vi "AlignDUT.vi"() -> ()   [LabVIEW 2018]
uses:
  <vilib>/userdefined/High Color/IMAQdx.ctl
  <vilib>/vision/driver/NI_Vision_Acquisition_Software.lvlib
  <vilib>/vision/NI_Vision_Development_Module.lvlib
panel:
  out "Average Length Between Fiducials":dbl format="%0.2f"
  in  "Number of Iterations":i32=50
  in  "Sensor Type":string(combo)="R0Hamamatsu"
  in  "Second Move OK?":bool
  in  "Second Fiducial OK?":bool
  in  "Second Fiducial in View?":bool
  in  "First Move OK?":bool
  in  "First Fiducial OK?":bool
  out "Pattern Matched Image":T1(plugin-control) caption="Template Image"
  out "Image Out":T1(plugin-control)
  in  "Fiducial 1":bool
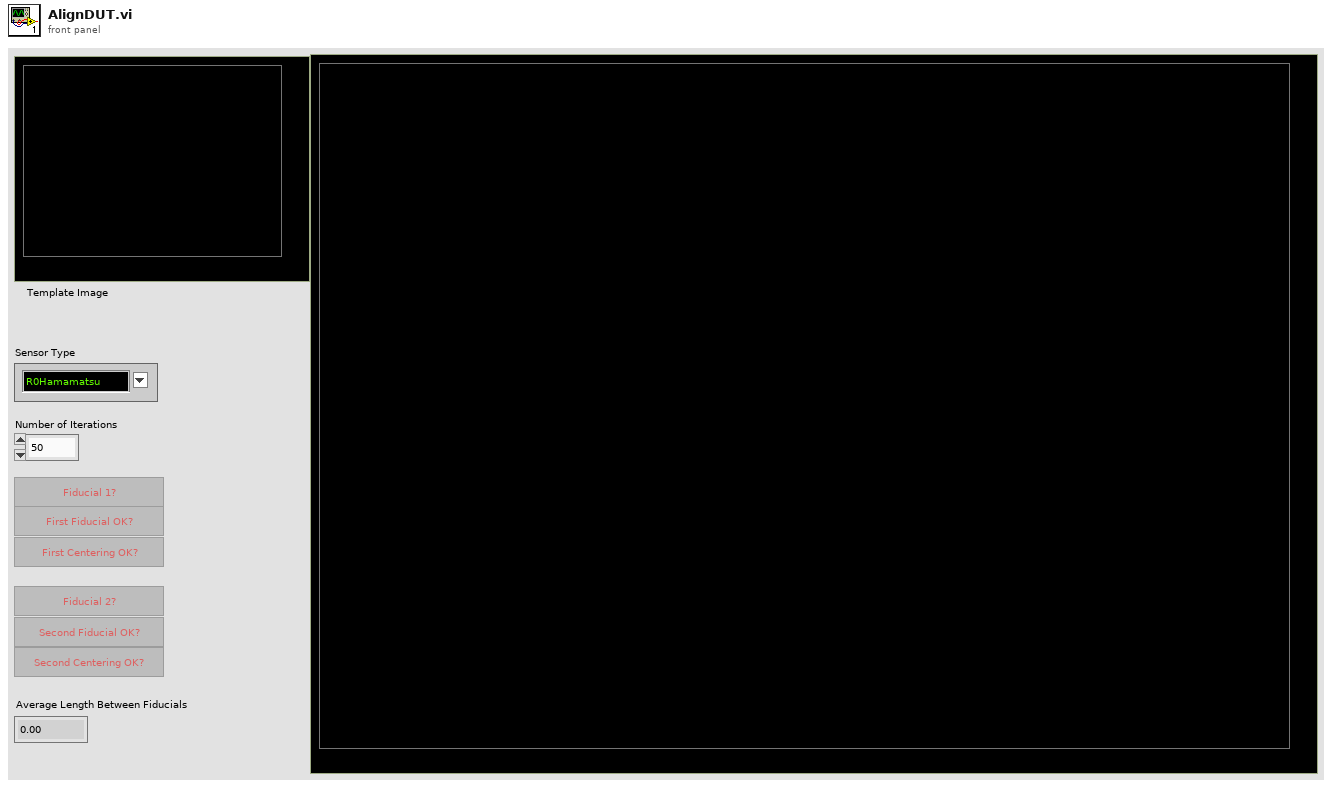
[diagram p1: front panel]
types:
  T1 = typedef "IMAQ Image.ctl" = refnum<image>
  T2 = enum8{"Enabled", "Disabled", "Disabled and Grayed Out"}
  T3 = typedef "Image Type" = u32
  T4 = typedef "IMAQdx.ctl" = refnum<k21>
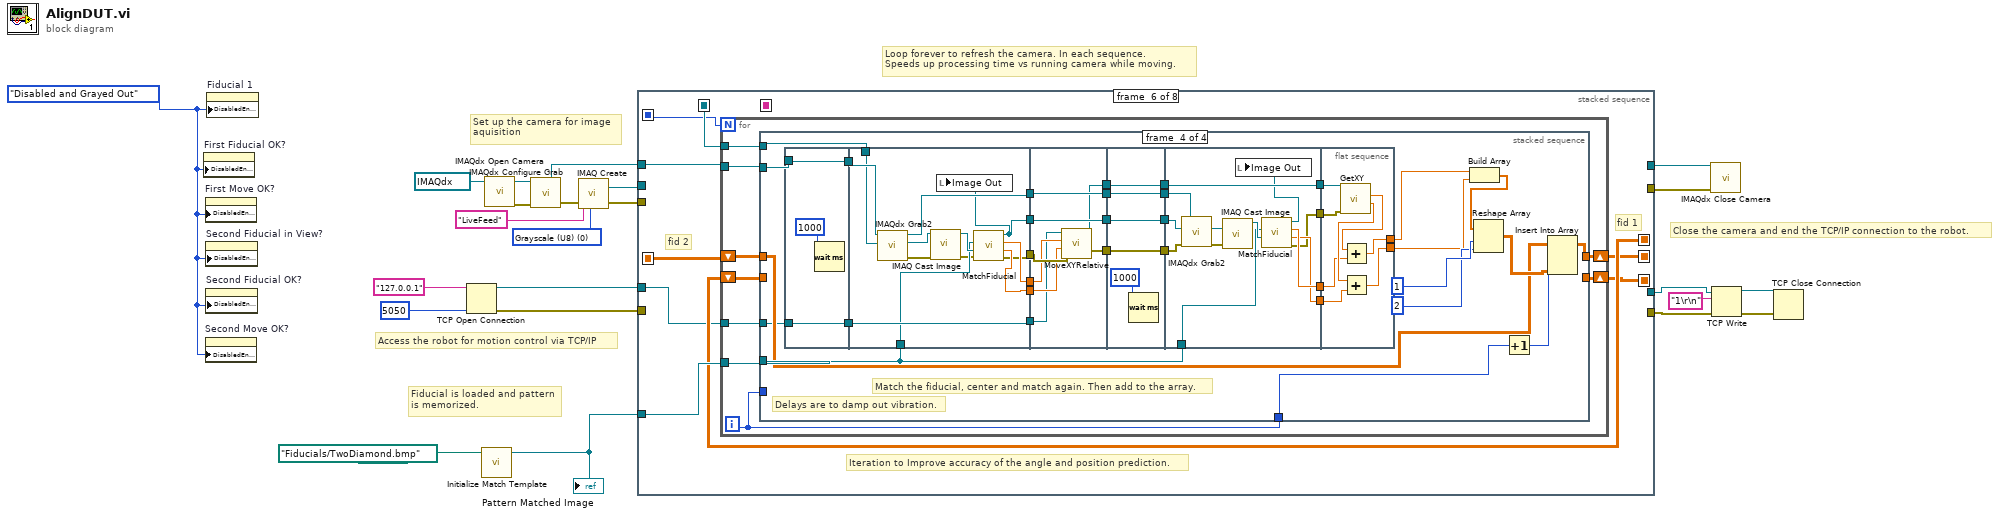
[diagram p0: block diagram]
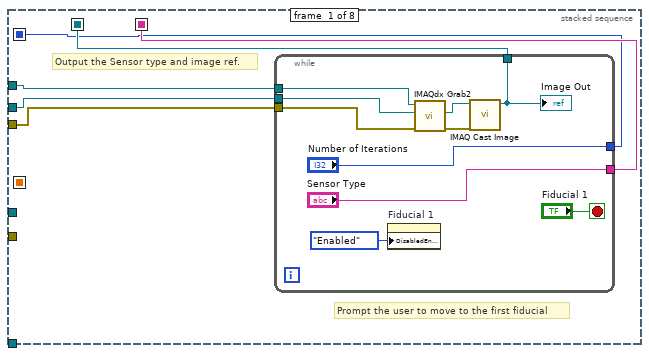
[diagram p2: hidden frame]
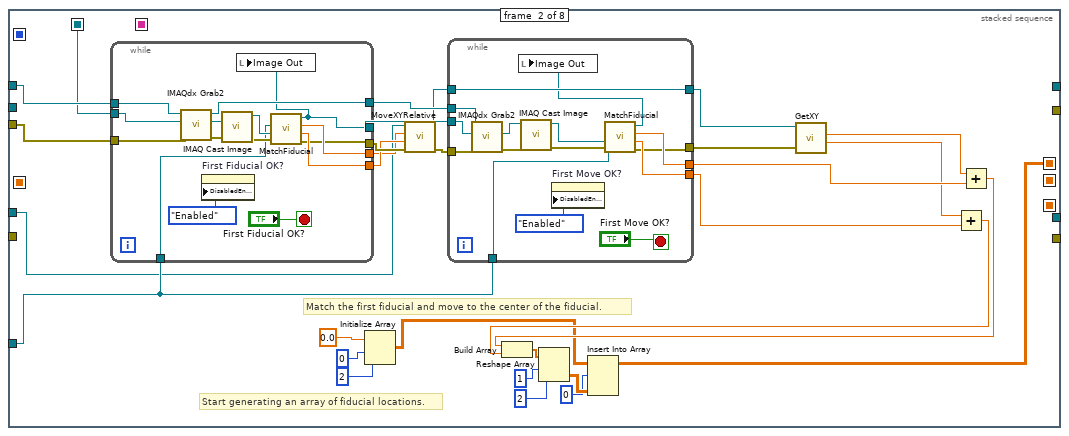
[diagram p3: hidden frame]
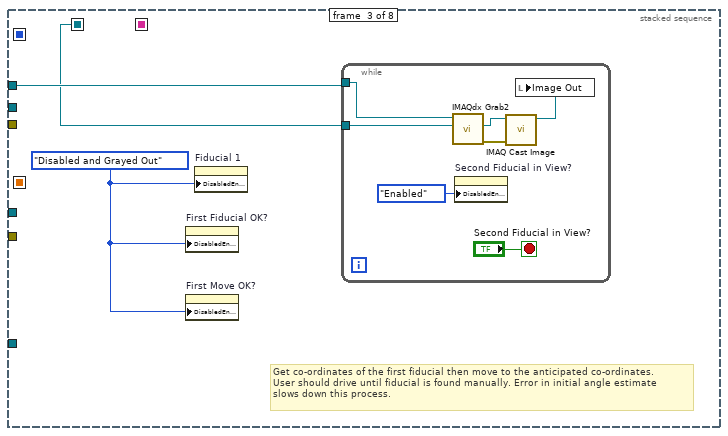
[diagram p4: hidden frame]
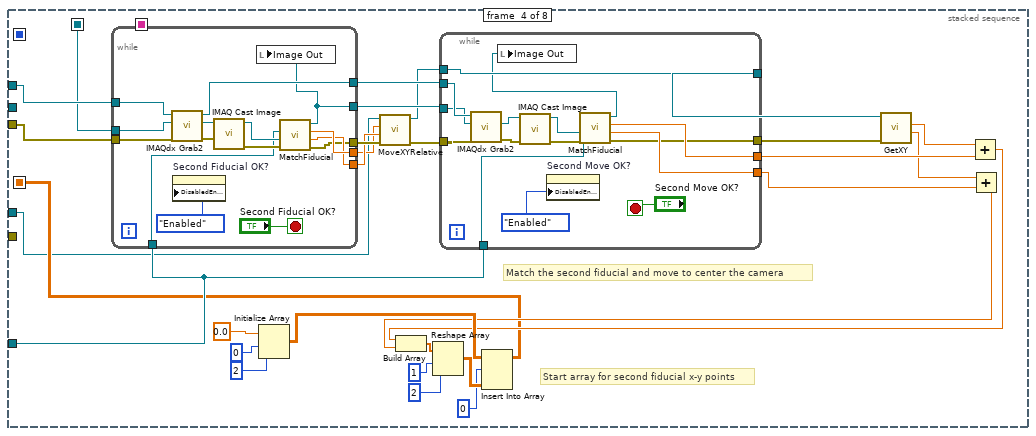
[diagram p5: hidden frame]
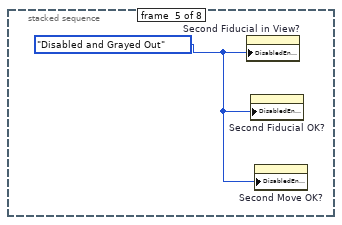
[diagram p6: hidden frame]
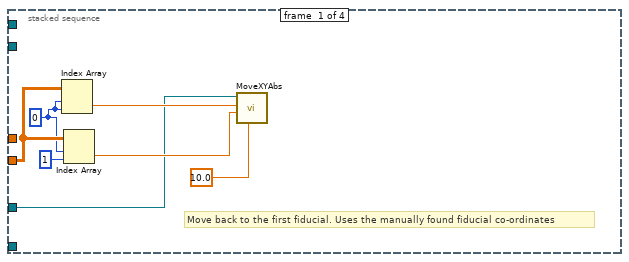
[diagram p7: hidden frame]
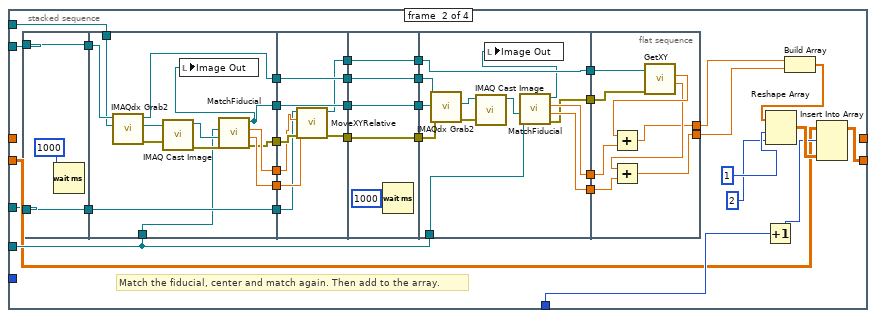
[diagram p8: hidden frame]
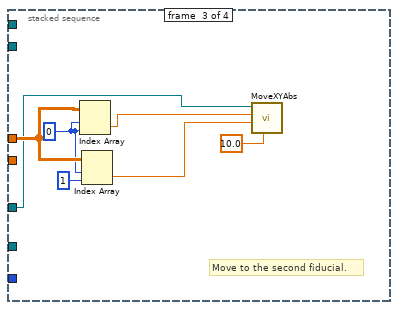
[diagram p9: hidden frame]
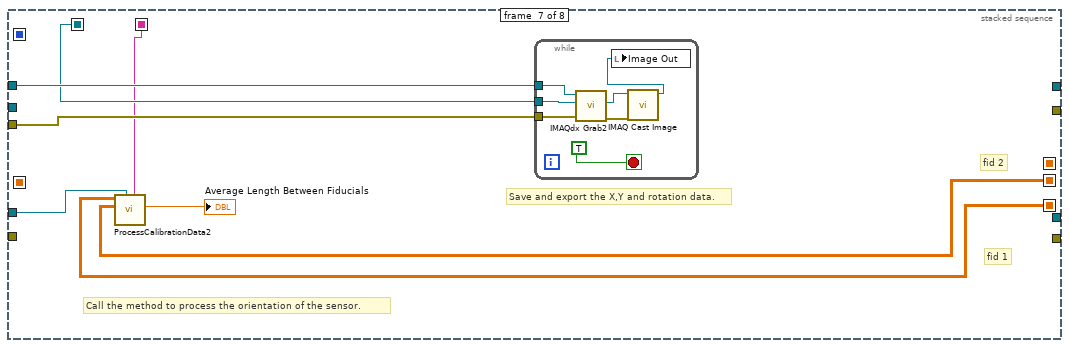
[diagram p10: hidden frame]
diagram:
  w1 = T2."Disabled and Grayed Out" ("Disabled")
  w12 = T3 0 items=["Grayscale (U8)", "Grayscale (I16)", "Grayscale (SGL)", "Complex (CSG)", "RGB (U32)", "HSL (U32)", "RGB (U64)", "Grayscale (U16)"] ("Image Type")
  # "Close the camera and end the TCP/IP connection to the robot."
  # "Access the robot for motion control via TCP/IP"
  # "Fiducial is loaded and pattern\nis memorized."
  # "Loop forever to refresh the camera. In each sequence. \nSpeeds up processing time vs running camera while moving."
  # "Set up the camera for image \naquisition"
  n1 = property on="First Fiducial OK?" class="Bool"("DisabledEnum"=w1) -> ()  [unwired: 2 in, 2 out]
  n2 = property on="First Move OK?" class="Bool"("DisabledEnum"=w1) -> ()  [unwired: 2 in, 2 out]
  n3 = property on="Second Move OK?" class="Bool"("DisabledEnum"=w1) -> ()  [unwired: 2 in, 2 out]
  n4 = property on="Second Fiducial in View?" class="Bool"("DisabledEnum"=w1) -> ()  [unwired: 2 in, 2 out]
  n5 = property on="Second Fiducial OK?" class="Bool"("DisabledEnum"=w1) -> ()  [unwired: 2 in, 2 out]
  n6 = property on="Fiducial 1" class="Bool"("DisabledEnum"=w1) -> ()  [unwired: 2 in, 2 out]
  n7 = TCP Open Connection(address="127.0.0.1", remote port or service name=u16 5050) -> (connection ID=w9:refnum<k5>, error out=w8:errorcluster)  [unwired: 3 in]
  n8 = call "Initialize Match Template.vi"("base path"=path "Fiducials/TwoDiamond.bmp") -> ("Pattern Matched Image"=w15:T1)  [unwired: 10 in]
  "Pattern Matched Image" <- w15
  n9 = call <vilib>:"IMAQdx Open Camera.vi"("Session In"=T4 "cam0") -> ("error out"=w21:errorcluster, "Session Out"=w22:T4)  [unwired: 9 in]
  n10 = call <vilib>:"IMAQdx Configure Grab.vi"("error in"=w21, "Session In"=w22) -> ("error out"=w19:errorcluster, "Session Out"=w18:T4)  [unwired: 8 in]
  n11 = call "IMAQ Create"("Image Name"="LiveFeed", "Image Type"=w12, "error in (no error)"=w19) -> ("New Image"=w17:T1, "error out"=w16:errorcluster)  [unwired: 2 in]
  n12 = stacked-sequence {
    seq-local: [_ _ _ w115 _ _ _ _] -> [_ _ _ _ _ w179 _ _]
    seq-local: [w26 _ _ _ _ _ _ _] -> [_ w62 w101 w133 _ w178 w374 _]
    seq-local: [_ w46 _ _ _ _ _ _] -> [_ _ _ _ _ w175 _ _]
    seq-local: [_ _ _ _ _ w173 _ _] -> [_ _ _ _ _ _ w373 _]
    seq-local: [_ _ _ _ _ w174 _ _] -> [_ _ _ _ _ _ w372 _]
    seq-local: [w25 _ _ _ _ _ _ _] -> [_ _ _ _ _ _ w370 _]
    seq-local: [w24 _ _ _ _ _ _ _] -> [_ _ _ _ _ w171 _ _]
    tunnel: w18 -> [w29 w68 w102 w134 _ w177 w376 w386]
    tunnel: w17 -> [w28 _ _ _ _ _ _ _]
    tunnel: w16 -> [w27 w64 _ w136 _ _ w375 w387]
    tunnel: w15 -> [_ w65 _ w135 _ w176 _ _]
    tunnel: [_ _ _ _ _ _ _ w387] -> w14
    tunnel: [_ _ _ _ _ _ _ w386] -> w13
    tunnel: w9 -> [_ w42 _ w112 _ w172 w371 w385]
    tunnel: [_ _ _ _ _ _ _ w385] -> w6
    tunnel: [_ _ _ _ _ _ _ w384] -> w7
    tunnel: w8 -> [_ _ _ _ _ _ _ w384]
    frame #0 {
      # "Output the Sensor type and image ref."
      # "Prompt the user to move to the first fiducial"
      n13 = while {
        tunnel: w29 -> [w38]
        tunnel: w27 -> [w37]
        tunnel: w28 -> [w36]
        tunnel: [w33] -> w26
        tunnel: ["Sensor Type"] -> w25
        tunnel: ["Number of Iterations"] -> w24
        stop <- "Fiducial 1" stop-if-true
        n14 = property on="Fiducial 1" class="Bool"("DisabledEnum"=T2."Enabled" ("Disabled")) -> ()  [unwired: 2 in, 2 out]
        n15 = call <vilib>:"IMAQdx Grab2.vi"("error in"=w37, "Image In"=w36, "Session In"=w38) -> ("error out"=w34:errorcluster, "Image Out"=w35:T1)  [unwired: 5 in, 2 out]
        n16 = call "IMAQ Cast Image"("error in (no error)"=w34, "Image Src"=w35) -> ("Image Dst Out"=w33:T1)  [unwired: 8 in, 1 out]
        "Image Out" <- w33
      }
    }
    frame #1 {
      # "Start generating an array of fiducial locations."
      # "Match the first fiducial and move to the center of the fiducial."
      n17 = while {
        tunnel: [w86] -> w63
        tunnel: [w99] -> w67
        tunnel: [w90] -> w69
        tunnel: w68 -> [w97]
        tunnel: w65 -> [w87]
        tunnel: w64 -> [w92]
        tunnel: [w96] -> w43
        tunnel: [w95] -> w44
        tunnel: w62 -> [w91]
        stop <- "First Fiducial OK?" stop-if-true
        n18 = call <vilib>:"IMAQdx Grab2.vi"("error in"=w92, "Image In"=w91, "Session In"=w97) -> ("error out"=w94:errorcluster, "Image Out"=w93:T1, "Session Out"=w99:T4)  [unwired: 5 in, 1 out]
        n19 = property on="First Fiducial OK?" class="Bool"("DisabledEnum"=T2."Enabled" ("Disabled")) -> ()  [unwired: 2 in, 2 out]
        n20 = call "IMAQ Cast Image"("error in (no error)"=w94, "Image Src"=w93) -> ("error out"=w89:errorcluster, "Image Dst Out"=w88:T1)  [unwired: 8 in]
        n21 = call "MatchFiducial.vi"("error in"=w89, "Image In"=w88, "Template Image"=w87) -> ("error out"=w90:errorcluster, "Y (um)"=w95:dbl, "X (um)"=w96:dbl, "Image Out"=w86:T1)  [unwired: 3 in, 2 out]
        n22 = local write "Image Out"(w86) -> ()
      }
      n23 = Initialize Array(0.0 ("element"), 0 ("dimension size"), 2 ("dimension size")) -> (w47:dbl[][])
      n24 = call "MoveXYRelative.vi"("error in (no error)"=w69, "Y"=w44, "X"=w43, "connection ID"=w42) -> ("error out"=w66:errorcluster, "connection ID 2"=w41:refnum<k5>)  [unwired: 6 in]
      n25 = while {
        tunnel: w67 -> [w83]
        tunnel: w66 -> [w76]
        tunnel: w65 -> [w71]
        tunnel: w63 -> [w77]
        tunnel: [w80] -> w55
        tunnel: [w79] -> w57
        tunnel: [w72] -> w58
        tunnel: w41 -> [w78]
        tunnel: [w78] -> w40
        stop <- "First Move OK?" stop-if-true
        n26 = call <vilib>:"IMAQdx Grab2.vi"("error in"=w76, "Image In"=w77, "Session In"=w83) -> ("error out"=w82:errorcluster, "Image Out"=w81:T1)  [unwired: 5 in, 2 out]
        n27 = call "IMAQ Cast Image"("error in (no error)"=w82, "Image Src"=w81) -> ("error out"=w75:errorcluster, "Image Dst Out"=w74:T1)  [unwired: 8 in]
        n28 = property on="First Move OK?" class="Bool"("DisabledEnum"=T2."Enabled" ("Disabled")) -> ()  [unwired: 2 in, 2 out]
        n29 = call "MatchFiducial.vi"("error in"=w75, "Image In"=w74, "Template Image"=w71) -> ("error out"=w72:errorcluster, "Y (um)"=w80:dbl, "X (um)"=w79:dbl, "Image Out"=w73:T1)  [unwired: 3 in, 2 out]
        n30 = local write "Image Out"(w73) -> ()
      }
      n31 = call "GetXY.vi"("error in (no error)"=w58, "connection ID"=w40) -> ("Y"=w54:dbl, "X"=w56:dbl)  [unwired: 6 in, 2 out]
      n32 = Add(x=w54, y=w55) -> (x+y=w48:dbl)
      n33 = Add(x=w56, y=w57) -> (x+y=w49:dbl)
      n34 = Build Array(w49, w48) -> (w53:dbl[])
      n35 = Reshape Array(w53, 1 ("dimension size"), 2 ("dimension size")) -> (w52:dbl[][])
      n36 = Insert Into Array(array=w47, index (row)=0, new element=w52) -> (w46:dbl[][])  [unwired: 1 in]
    }
    frame #2 {
      w100 = T2."Disabled and Grayed Out" ("Disabled")
      # "Get co-ordinates of the first fiducial then move to the anticipated co-ordinates. \nUser should drive until fiducial is found manually. Error in initial angle estimate \nslows down this process."
      n37 = property on="First Fiducial OK?" class="Bool"("DisabledEnum"=w100) -> ()  [unwired: 2 in, 2 out]
      n38 = property on="First Move OK?" class="Bool"("DisabledEnum"=w100) -> ()  [unwired: 2 in, 2 out]
      n39 = property on="Fiducial 1" class="Bool"("DisabledEnum"=w100) -> ()  [unwired: 2 in, 2 out]
      n40 = while {
        tunnel: w101 -> [w108]
        tunnel: w102 -> [w107]
        stop <- "Second Fiducial in View?" stop-if-true
        n41 = call <vilib>:"IMAQdx Grab2.vi"("Image In"=w108, "Session In"=w107) -> ("error out"=w106:errorcluster, "Image Out"=w105:T1)  [unwired: 6 in, 2 out]
        n42 = property on="Second Fiducial in View?" class="Bool"("DisabledEnum"=T2."Enabled" ("Disabled")) -> ()  [unwired: 2 in, 2 out]
        n43 = call "IMAQ Cast Image"("error in (no error)"=w106, "Image Src"=w105) -> ("Image Dst Out"=w104:T1)  [unwired: 8 in, 1 out]
        n44 = local write "Image Out"(w104) -> ()
      }
    }
    frame #3 {
      # "Start array for second fiducial x-y points"
      # "Match the second fiducial and move to center the camera"
      n45 = while {
        tunnel: [w160] -> w138
        tunnel: [w161] -> w137
        tunnel: w134 -> [w168]
        tunnel: w135 -> [w157]
        tunnel: w136 -> [w162]
        tunnel: w133 -> [w163]
        tunnel: [w167] -> w113
        tunnel: [w166] -> w114
        tunnel: [w156] -> w132
        stop <- "Second Fiducial OK?" stop-if-true
        n46 = call <vilib>:"IMAQdx Grab2.vi"("error in"=w162, "Image In"=w163, "Session In"=w168) -> ("error out"=w165:errorcluster, "Image Out"=w164:T1, "Session Out"=w160:T4)  [unwired: 5 in, 1 out]
        n47 = property on="Second Fiducial OK?" class="Bool"("DisabledEnum"=T2."Enabled" ("Disabled")) -> ()  [unwired: 2 in, 2 out]
        n48 = call "IMAQ Cast Image"("error in (no error)"=w165, "Image Src"=w164) -> ("error out"=w158:errorcluster, "Image Dst Out"=w159:T1)  [unwired: 8 in]
        n49 = call "MatchFiducial.vi"("error in"=w158, "Image In"=w159, "Template Image"=w157) -> ("error out"=w161:errorcluster, "Y (um)"=w166:dbl, "X (um)"=w167:dbl, "Image Out"=w156:T1)  [unwired: 3 in, 2 out]
        n50 = local write "Image Out"(w156) -> ()
      }
      n51 = Initialize Array(0.0 ("element"), 0 ("dimension size"), 2 ("dimension size")) -> (w119:dbl[][])
      n52 = call "MoveXYRelative.vi"("error in (no error)"=w137, "Y"=w114, "X"=w113, "connection ID"=w112) -> ("error out"=w139:errorcluster, "connection ID 2"=w111:refnum<k5>)  [unwired: 6 in]
      n53 = while {
        tunnel: w138 -> [w153]
        tunnel: w139 -> [w146]
        tunnel: w135 -> [w143]
        tunnel: w132 -> [w147]
        tunnel: [w150] -> w130
        tunnel: [w149] -> w128
        tunnel: [w141] -> w127
        tunnel: w111 -> [w148]
        tunnel: [w148] -> w110
        stop <- "Second Move OK?" stop-if-true
        n54 = call <vilib>:"IMAQdx Grab2.vi"("error in"=w146, "Image In"=w147, "Session In"=w153) -> ("error out"=w152:errorcluster, "Image Out"=w151:T1)  [unwired: 5 in, 2 out]
        n55 = call "IMAQ Cast Image"("error in (no error)"=w152, "Image Src"=w151) -> ("error out"=w145:errorcluster, "Image Dst Out"=w144:T1)  [unwired: 8 in]
        n56 = property on="Second Move OK?" class="Bool"("DisabledEnum"=T2."Enabled" ("Disabled")) -> ()  [unwired: 2 in, 2 out]
        n57 = call "MatchFiducial.vi"("error in"=w145, "Image In"=w144, "Template Image"=w143) -> ("error out"=w141:errorcluster, "Y (um)"=w149:dbl, "X (um)"=w150:dbl, "Image Out"=w142:T1)  [unwired: 3 in, 2 out]
        n58 = local write "Image Out"(w142) -> ()
      }
      n59 = call "GetXY.vi"("error in (no error)"=w127, "connection ID"=w110) -> ("Y"=w129:dbl, "X"=w131:dbl)  [unwired: 6 in, 2 out]
      n60 = Add(x=w131, y=w130) -> (x+y=w117:dbl)
      n61 = Add(x=w129, y=w128) -> (x+y=w116:dbl)
      n62 = Build Array(w117, w116) -> (w123:dbl[])
      n63 = Reshape Array(w123, 1 ("dimension size"), 2 ("dimension size")) -> (w122:dbl[][])
      n64 = Insert Into Array(array=w119, index (row)=0, new element=w122) -> (w115:dbl[][])  [unwired: 1 in]
    }
    frame #4 {
      w170 = T2."Disabled and Grayed Out" ("Disabled")
      n65 = property on="Second Fiducial in View?" class="Bool"("DisabledEnum"=w170) -> ()  [unwired: 2 in, 2 out]
      n66 = property on="Second Fiducial OK?" class="Bool"("DisabledEnum"=w170) -> ()  [unwired: 2 in, 2 out]
      n67 = property on="Second Move OK?" class="Bool"("DisabledEnum"=w170) -> ()  [unwired: 2 in, 2 out]
    }
    frame #5 {
      # "fid 1"
      # "fid 2"
      # "Iteration to Improve accuracy of the angle and position prediction."
      n68 = for {
        N: w171 -> [_]
        tunnel: w178 -> [w186]
        tunnel: w177 -> [w185]
        tunnel: w176 -> [w187]
        shift-right: [w182] -> w173
        shift-left: w179 -> [w188]
        shift-right: [w183] -> w174
        shift-left: w175 -> [w184]
        tunnel: w172 -> [w181]
        i -> [w180]
        n69 = stacked-sequence {
          tunnel: w188 -> [_ _ w284 w304]
          tunnel: w187 -> [_ w227 _ w288]
          tunnel: w180 -> [_ w219 _ w307]
          tunnel: w186 -> [_ w216 _ w305]
          tunnel: w185 -> [_ w217 _ w306]
          tunnel: w184 -> [w194 w215 _ _]
          tunnel: [_ w214 _ _] -> w183
          tunnel: [_ _ _ w303] -> w182
          tunnel: w181 -> [w190 w210 w280 w300]
          tunnel: w180 -> [_ _ _ _]
          frame #0 {
            w193 = 0 ("index (row)")
            # "Move back to the first fiducial. Uses the manually found fiducial co-ordinates"
            n70 = Index Array(array=w194, index (row)=w193, index (col)=w193) -> (element=w191:dbl)
            n71 = Index Array(array=w194, index (row)=w193, index (col)=1) -> (element=w192:dbl)
            n72 = call "MoveXYAbs.vi"("%Speed"=10.0, "Y"=w192, "X"=w191, "connection ID 2"=w190) -> ()  [unwired: 6 in, 2 out]
          }
          frame #1 {
            # "Match the fiducial, center and match again. Then add to the array."
            n73 = flat-sequence {
              tunnel: w210 -> [w231]
              tunnel: w217 -> [w232]
              tunnel: [w232] -> w200
              tunnel: [w231] -> w199
              tunnel: w227 -> [w234]
              tunnel: [w236] -> w229
              tunnel: [w242] -> w228
              tunnel: w216 -> [w238]
              tunnel: [w241] -> w213
              tunnel: [w240] -> w212
              tunnel: [w239] -> w211
              tunnel: w200 -> [w243]
              tunnel: w199 -> [w239]
              tunnel: [w233] -> w198
              tunnel: w229 -> [w251]
              tunnel: w228 -> [w253]
              tunnel: [w253] -> w208
              tunnel: [w252] -> w206
              tunnel: [w250] -> w204
              tunnel: w213 -> [w248]
              tunnel: w212 -> [w249]
              tunnel: w211 -> [w247]
              tunnel: [w246] -> w202
              tunnel: w198 -> [w252]
              tunnel: w208 -> [w258]
              tunnel: [w258] -> w207
              tunnel: w206 -> [w257]
              tunnel: [w257] -> w205
              tunnel: w204 -> [w256]
              tunnel: [w256] -> w203
              tunnel: w202 -> [w255]
              tunnel: [w255] -> w201
              tunnel: w207 -> [w268]
              tunnel: w205 -> [w259]
              tunnel: w203 -> [w264]
              tunnel: w227 -> [w261]
              tunnel: [w263] -> w226
              tunnel: [w267] -> w224
              tunnel: [w266] -> w223
              tunnel: [w265] -> w209
              tunnel: w201 -> [w265]
              tunnel: w226 -> [w278]
              tunnel: w224 -> [w275]
              tunnel: w223 -> [w274]
              tunnel: [w273] -> w197
              tunnel: [w272] -> w196
              tunnel: w209 -> [w271]
              frame #0 {
                n74 = Wait (ms)(milliseconds to wait=u32 1000) -> ()  [unwired: 1 out]
              }
              frame #1 {
                n75 = call <vilib>:"IMAQdx Grab2.vi"("Image In"=w238, "Session In"=w243) -> ("error out"=w245:errorcluster, "Image Out"=w244:T1, "Session Out"=w242:T4)  [unwired: 6 in, 1 out]
                n76 = call "IMAQ Cast Image"("error in (no error)"=w245, "Image Src"=w244) -> ("error out"=w237:errorcluster, "Image Dst Out"=w235:T1)  [unwired: 8 in]
                n77 = call "MatchFiducial.vi"("error in"=w237, "Image In"=w235, "Template Image"=w234) -> ("error out"=w236:errorcluster, "Y (um)"=w240:dbl, "X (um)"=w241:dbl, "Image Out"=w233:T1)  [unwired: 3 in, 2 out]
                n78 = local write "Image Out"(w233) -> ()
              }
              frame #2 {
                n79 = call "MoveXYRelative.vi"("error in (no error)"=w251, "Y"=w249, "X"=w248, "connection ID"=w247) -> ("error out"=w250:errorcluster, "connection ID 2"=w246:refnum<k5>)  [unwired: 6 in]
              }
              frame #3 {
                n80 = Wait (ms)(milliseconds to wait=u32 1000) -> ()  [unwired: 1 out]
              }
              frame #4 {
                n81 = call <vilib>:"IMAQdx Grab2.vi"("error in"=w264, "Image In"=w259, "Session In"=w268) -> ("error out"=w269:errorcluster, "Image Out"=w270:T1)  [unwired: 5 in, 2 out]
                n82 = call "IMAQ Cast Image"("error in (no error)"=w269, "Image Src"=w270) -> ("Image Dst Out"=w262:T1)  [unwired: 8 in, 1 out]
                n83 = call "MatchFiducial.vi"("Image In"=w262, "Template Image"=w261) -> ("error out"=w263:errorcluster, "Y (um)"=w266:dbl, "X (um)"=w267:dbl, "Image Out"=w260:T1)  [unwired: 4 in, 2 out]
                n84 = local write "Image Out"(w260) -> ()
              }
              frame #5 {
                n85 = call "GetXY.vi"("error in (no error)"=w278, "connection ID"=w271) -> ("Y"=w276:dbl, "X"=w277:dbl)  [unwired: 6 in, 2 out]
                n86 = Add(x=w277, y=w275) -> (x+y=w273:dbl)
                n87 = Add(x=w276, y=w274) -> (x+y=w272:dbl)
              }
            }
            n88 = Increment(x=w219) -> (x+1=w218:i32)
            n89 = Build Array(w197, w196) -> (w222:dbl[])
            n90 = Reshape Array(w222, 1 ("dimension size"), 2 ("dimension size")) -> (w225:dbl[][])
            n91 = Insert Into Array(array=w215, index (row)=w218, new element=w225) -> (w214:dbl[][])  [unwired: 1 in]
          }
          frame #2 {
            w283 = 0 ("index (row)")
            # "Move to the second fiducial."
            n92 = Index Array(array=w284, index (row)=w283, index (col)=w283) -> (element=w282:dbl)
            n93 = Index Array(array=w284, index (row)=w283, index (col)=1) -> (element=w281:dbl)
            n94 = call "MoveXYAbs.vi"("%Speed"=10.0, "Y"=w281, "X"=w282, "connection ID 2"=w280) -> ()  [unwired: 6 in, 2 out]
          }
          frame #3 {
            # "Delays are to damp out vibration."
            # "Match the fiducial, center and match again. Then add to the array."
            n95 = flat-sequence {
              tunnel: w300 -> [w321]
              tunnel: w306 -> [w322]
              tunnel: [w322] -> w290
              tunnel: [w321] -> w289
              tunnel: w288 -> [w326]
              tunnel: [w332] -> w319
              tunnel: [w323] -> w318
              tunnel: [w328] -> w317
              tunnel: [w325] -> w316
              tunnel: w305 -> [w329]
              tunnel: [w331] -> w302
              tunnel: [w330] -> w301
              tunnel: w290 -> [w333]
              tunnel: w289 -> [w330]
              tunnel: w319 -> [w338]
              tunnel: w318 -> [w341]
              tunnel: w317 -> [w343]
              tunnel: w316 -> [w342]
              tunnel: [w343] -> w298
              tunnel: [w342] -> w296
              tunnel: [w340] -> w294
              tunnel: w302 -> [w339]
              tunnel: w301 -> [w337]
              tunnel: [w336] -> w292
              tunnel: w298 -> [w348]
              tunnel: [w348] -> w297
              tunnel: w296 -> [w347]
              tunnel: [w347] -> w295
              tunnel: w294 -> [w346]
              tunnel: [w346] -> w293
              tunnel: w292 -> [w345]
              tunnel: [w345] -> w291
              tunnel: w297 -> [w358]
              tunnel: w295 -> [w354]
              tunnel: w293 -> [w353]
              tunnel: w288 -> [w351]
              tunnel: [w349] -> w315
              tunnel: [w357] -> w314
              tunnel: [w356] -> w313
              tunnel: [w355] -> w299
              tunnel: w291 -> [w355]
              tunnel: w315 -> [w368]
              tunnel: w314 -> [w365]
              tunnel: w313 -> [w364]
              tunnel: [w363] -> w287
              tunnel: [w362] -> w286
              tunnel: w299 -> [w361]
              frame #0 {
                n96 = Wait (ms)(milliseconds to wait=u32 1000) -> ()  [unwired: 1 out]
              }
              frame #1 {
                n97 = call <vilib>:"IMAQdx Grab2.vi"("Image In"=w329, "Session In"=w333) -> ("error out"=w335:errorcluster, "Image Out"=w334:T1, "Session Out"=w328:T4)  [unwired: 6 in, 1 out]
                n98 = call "IMAQ Cast Image"("error in (no error)"=w335, "Image Src"=w334) -> ("error out"=w324:errorcluster, "Image Dst Out"=w327:T1)  [unwired: 8 in]
                n99 = call "MatchFiducial.vi"("error in"=w324, "Image In"=w327, "Template Image"=w326) -> ("error out"=w323:errorcluster, "Y (um)"=w332:dbl, "X (um)"=w331:dbl, "Image Out"=w325:T1)  [unwired: 3 in, 2 out]
                n100 = local write "Image Out"(w325) -> ()
              }
              frame #2 {
                n101 = call "MoveXYRelative.vi"("error in (no error)"=w341, "Y"=w338, "X"=w339, "connection ID"=w337) -> ("error out"=w340:errorcluster, "connection ID 2"=w336:refnum<k5>)  [unwired: 6 in]
              }
              frame #3 {
                n102 = Wait (ms)(milliseconds to wait=u32 1000) -> ()  [unwired: 1 out]
              }
              frame #4 {
                n103 = call <vilib>:"IMAQdx Grab2.vi"("error in"=w353, "Image In"=w354, "Session In"=w358) -> ("error out"=w359:errorcluster, "Image Out"=w360:T1)  [unwired: 5 in, 2 out]
                n104 = call "IMAQ Cast Image"("error in (no error)"=w359, "Image Src"=w360) -> ("Image Dst Out"=w352:T1)  [unwired: 8 in, 1 out]
                n105 = call "MatchFiducial.vi"("Image In"=w352, "Template Image"=w351) -> ("error out"=w349:errorcluster, "Y (um)"=w356:dbl, "X (um)"=w357:dbl, "Image Out"=w350:T1)  [unwired: 4 in, 2 out]
                n106 = local write "Image Out"(w350) -> ()
              }
              frame #5 {
                n107 = call "GetXY.vi"("error in (no error)"=w368, "connection ID"=w361) -> ("Y"=w366:dbl, "X"=w367:dbl)  [unwired: 6 in, 2 out]
                n108 = Add(x=w367, y=w365) -> (x+y=w363:dbl)
                n109 = Add(x=w366, y=w364) -> (x+y=w362:dbl)
              }
            }
            n110 = Build Array(w287, w286) -> (w311:dbl[])
            n111 = Reshape Array(w311, 1 ("dimension size"), 2 ("dimension size")) -> (w312:dbl[][])
            n112 = Increment(x=w307) -> (x+1=w308:i32)
            n113 = Insert Into Array(array=w304, index (row)=w308, new element=w312) -> (w303:dbl[][])  [unwired: 1 in]
          }
        }
      }
    }
    frame #6 {
      # "Call the method to process the orientation of the sensor."
      # "fid 2"
      # "fid 1"
      # "Save and export the X,Y and rotation data."
      n114 = call "ProcessCalibrationData2.vi"("Sensor Type"=w370, "connection ID"=w371, "Fiducial 2"=w373, "Fiducial 1"=w372) -> ("Avg Length"=→"Average Length Between Fiducials":dbl)  [unwired: 7 in]
      n115 = while {
        tunnel: w376 -> [w383]
        tunnel: w374 -> [w382]
        tunnel: w375 -> [w381]
        stop <- TRUE ("Computation OK?") stop-if-true
        n116 = call <vilib>:"IMAQdx Grab2.vi"("error in"=w381, "Image In"=w382, "Session In"=w383) -> ("error out"=w380:errorcluster, "Image Out"=w379:T1)  [unwired: 5 in, 2 out]
        n117 = call "IMAQ Cast Image"("error in (no error)"=w380, "Image Src"=w379) -> ("Image Dst Out"=w378:T1)  [unwired: 8 in, 1 out]
        n118 = local write "Image Out"(w378) -> ()
      }
    }
    frame #7 {
      # "Close connections"
    }
  }
  n119 = call <vilib>:"IMAQdx Close Camera.vi"("error in"=w14, "Session In"=w13) -> ()  [unwired: 9 in, 1 out]
  n120 = TCP Write(connection ID=w6, data in="1\r\n", error in (no error)=w7) -> (connection ID out=w4:refnum<k5>, error out=w5:errorcluster)  [unwired: 1 in, 1 out]
  n121 = TCP Close Connection(connection ID=w4, error in (no error)=w5) -> ()  [unwired: 1 in, 2 out]
